vi "Destroy Config.vi"(8 "error in":errorcluster) -> (0 "error out":errorcluster)   [LabVIEW 2020, in "Configuration.lvclass"]
doc: "Remove this module's config from the DCFG UI.\n____\nPeloton Config 2.0.0.9\nCopyright (c) 2024, Peloton"
uses:
  Configuration.lvclass
  <vilib>/Peloton/Peloton Config/DCFG Framework/Peloton_lib_DCFG Framework.lvlib
  CML UI.lvlib
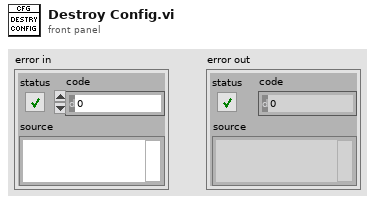
[diagram p1: front panel]
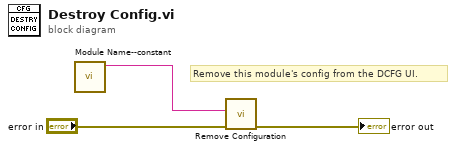
[diagram p0: block diagram]
diagram:
  # "Remove this module's config from the DCFG UI."
  n1 = call "Module Name--constant.vi"() -> ("Module Name"=w1:string)  [unwired: 11 in]
  n2 = call <vilib>:"Remove Configuration.vi"("error in"="error in", "Config Name"=w1) -> ("error out"=→"error out":errorcluster)  [unwired: 9 in]
